vi "Shutdown Camera.vi"(8 "error in (no error)":errorcluster, 11 "CCDCamera in":refnum<class "Sim_Ixon_Ultra.lvclass">) -> (0 "error out":errorcluster, 3 "CCDCamera out":refnum<class "Sim_Ixon_Ultra.lvclass">)   [LabVIEW 2018, in "Sim_Ixon_Ultra.lvclass"]
doc: "Shut down the camera"
uses:
  Sim_Ixon_Ultra.lvclass
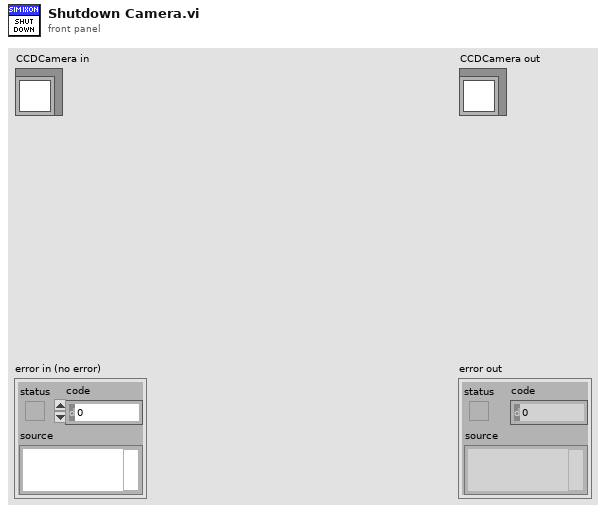
[diagram p1: front panel]
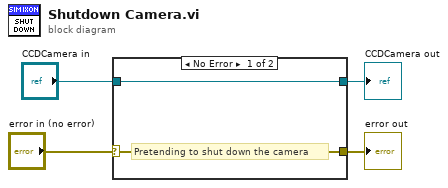
[diagram p0: block diagram]
diagram:
  n1 = case shown="No Error" "error in (no error)" {
    selector: "error in (no error)" -> [w5 w8]
    tunnel: [w5 w8] -> w3
    tunnel: [w6 w7] -> w1
    tunnel: "CCDCamera in" -> [w6 w7]
    frame No Error {
      # "Pretending to shut down the camera"
    }
    frame Error {
    }
  }
  "error out" <- w3
  "CCDCamera out" <- w1
